vi "SpectraBinning.vi"(4 "BinType":T1, 5 "BinWidth":dbl=1.0, 7 "Binning":bool=TRUE, 8 "error in (no error)":errorcluster, 9 "Signal":dbl[](array[numeric]), 10 "m/z Array":dbl[](array[numeric]), 11 "GraphsRef.":refnum<vi>) -> (0 "error out":errorcluster, 2 "BinnedSpectrum":cluster{"m/z Array":dbl[], "Signal":dbl[]})   [LabVIEW 2012]
uses:
  BinType.ctl
  <vilib>/Analysis/baseanly.llb/Mean (DBL).vi
  <vilib>/Analysis/NI_AALBase.lvlib
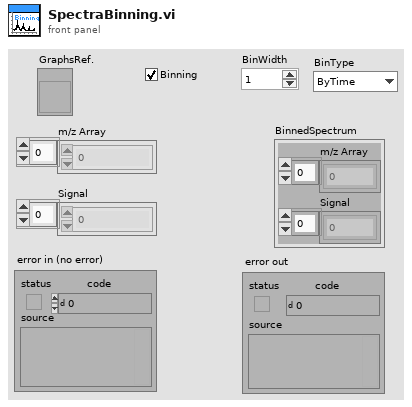
[diagram p1: front panel]
types:
  T1 = typedef "BinType.ctl" = enum16{"ByTime", "ByScreen", "ByMass", "ToUnitMass"}
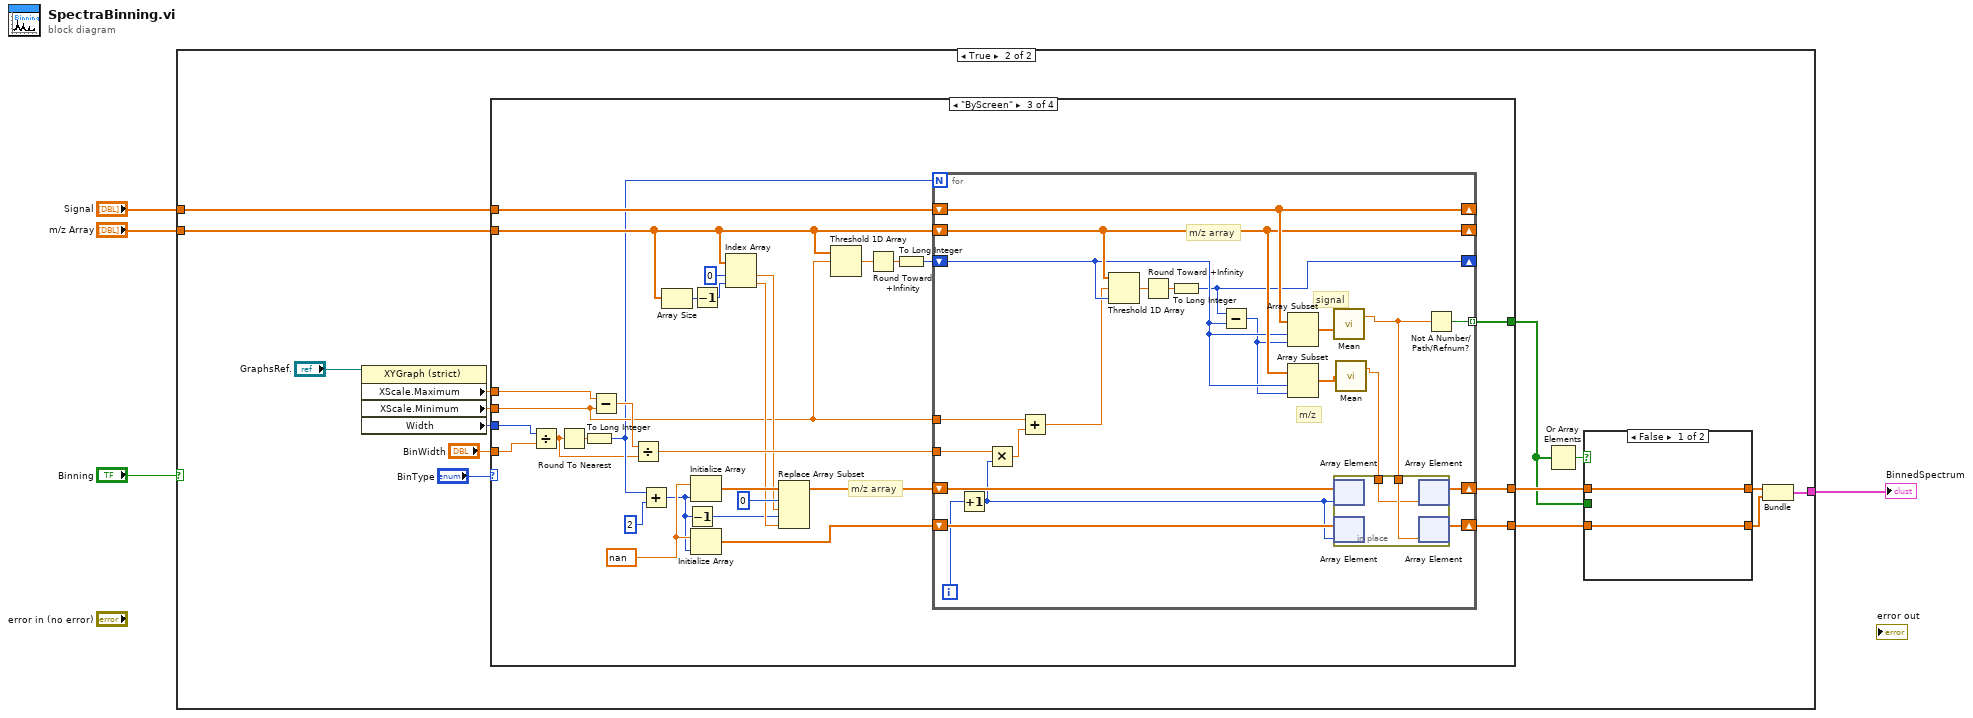
[diagram p0: block diagram]
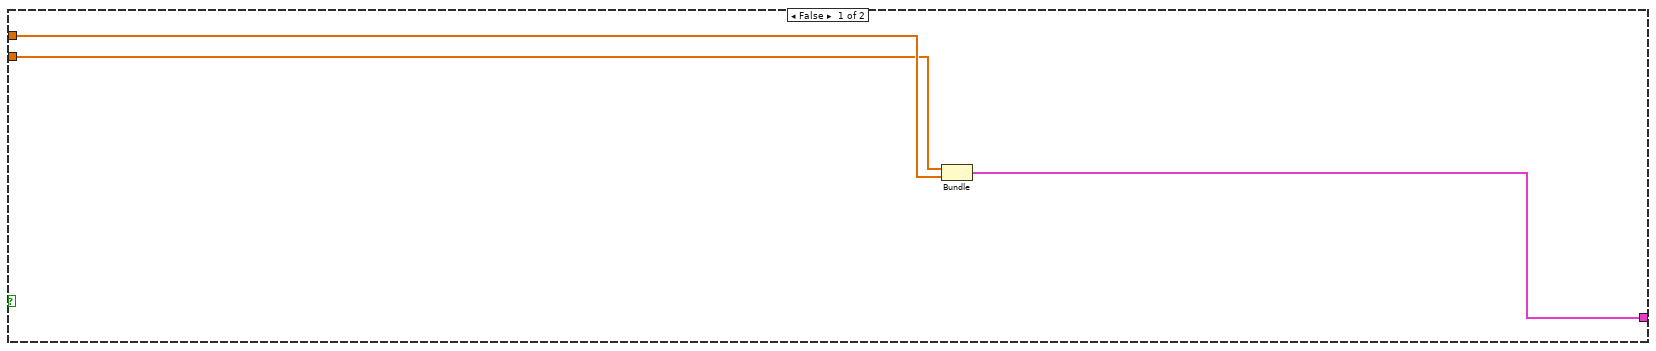
[diagram p2: hidden frame]
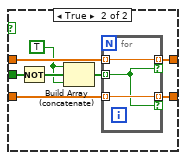
[diagram p3: hidden frame]
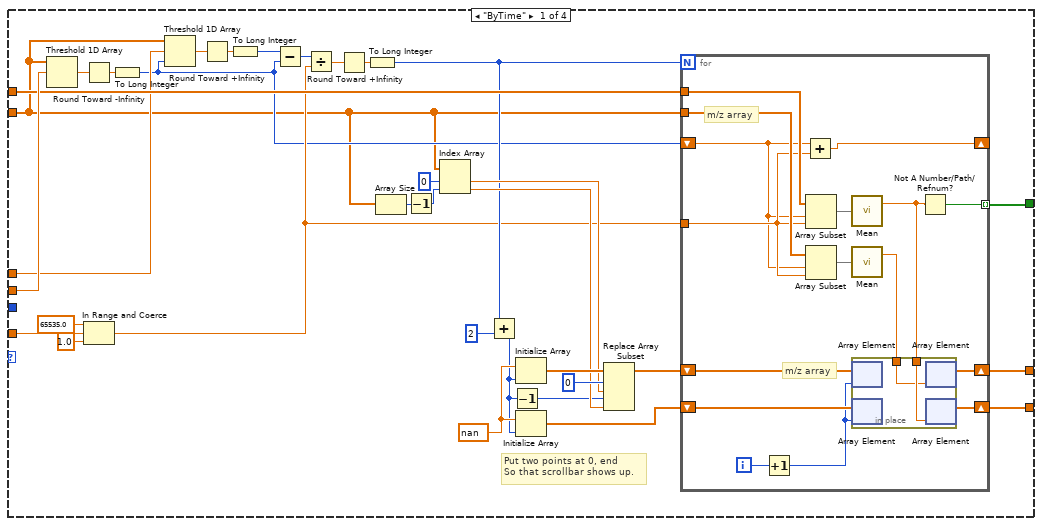
[diagram p4: hidden frame]
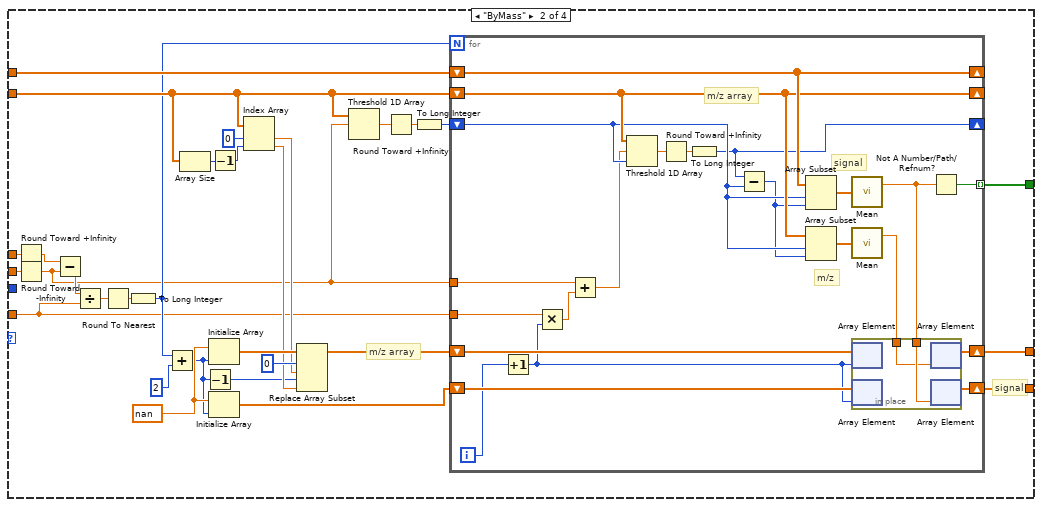
[diagram p5: hidden frame]
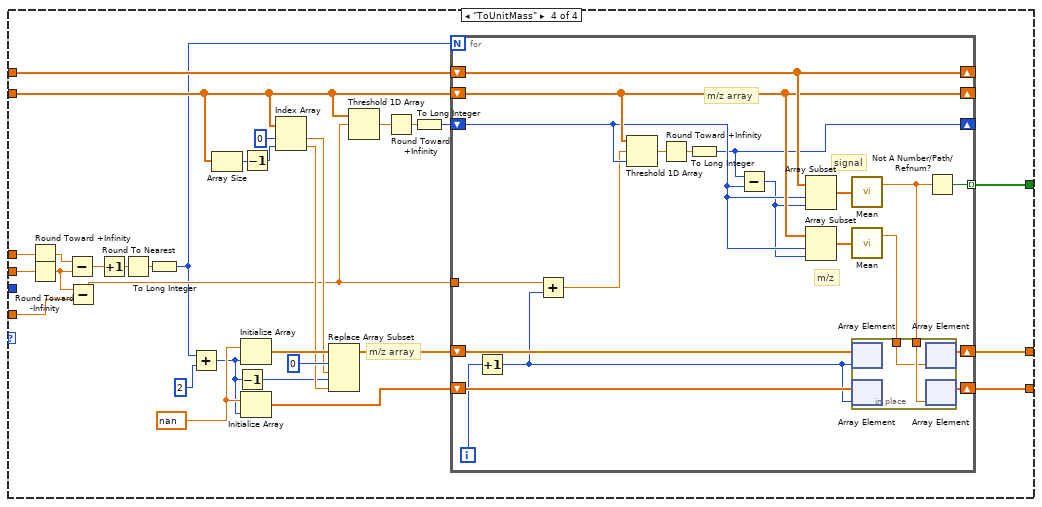
[diagram p6: hidden frame]
diagram:
  n1 = case shown="True" "Binning" {
    tunnel: [w7 w20] -> w4
    tunnel: "Signal" -> [w6 w10]
    tunnel: "m/z Array" -> [w5 w9]
    frame False {
      n2 = Bundle("m/z Array"=w5, "Signal"=w6) -> (w7:cluster{"m/z Array":dbl[], "Signal":dbl[]})  [unwired: 1 in]
    }
    frame True {
      n3 = property class="XYGraph (strict)"(reference="GraphsRef.") -> ("XScale.Maximum"=w13:dbl, "XScale.Minimum"=w12:dbl, "Width"=w11:u32)  [unwired: 1 in, 2 out]
      n4 = case shown="\"ByScreen\"" "BinType" {
        tunnel: w10 -> [w55 w117 w171 w226]
        tunnel: w9 -> [w36 w108 w160 w217]
        tunnel: w13 -> [w40 w102 w154 w211]
        tunnel: w12 -> [w56 w99 w150 w207]
        tunnel: w11 -> [_ _ w147 _]
        tunnel: "BinWidth" -> [w50 w95 w146 w199]
        tunnel: [w42 w90 w143 w197] -> w18
        tunnel: [w43 w89 w144 w198] -> w17
        tunnel: [w41 w91 w142 w196] -> w16
        frame "ByTime" {
          w67 = nan ("x/y")
          # "Put two points at 0, end\nSo that scrollbar shows up."
          n5 = Threshold 1D Array(2:w56, 3:w36) -> (0:w69:dbl)  [unwired: 1 in]
          n6 = Round Toward -Infinity(1:w69) -> (0:w68:dbl)
          n7 = In Range and Coerce(upper limit=65535.0, x=w50, lower limit=1.0) -> (coerced(x)=w46:dbl)  [unwired: 1 out]
          n8 = To Long Integer(number=w68) -> (32bit integer=w39:i32)
          n9 = Threshold 1D Array(1:w39, 2:w40, 3:w36) -> (0:w53:dbl)
          n10 = Round Toward +Infinity(x=w53) -> (ceil(x): smallest int >= x=w54:dbl)
          n11 = To Long Integer(number=w54) -> (32bit integer=w52:i32)
          n12 = Subtract(x=w52, y=w39) -> (x-y=w51:i32)
          n13 = Divide(x=w51, y=w46) -> (x/y=w48:dbl)
          n14 = Round Toward +Infinity(x=w48) -> (ceil(x): smallest int >= x=w49:dbl)
          n15 = To Long Integer(number=w49) -> (32bit integer=w47:i32)
          n16 = Array Size(array=w36) -> (size(s)=w59:i32)
          n17 = Decrement(x=w59) -> (x-1=w57:i32)
          n18 = Index Array(array=w36, index #1=0 ("index"), index #2=w57) -> (element #1=w61:dbl, element #2=w60:dbl)
          n19 = Add(x=w47, y=2) -> (x+y=w38:i32)
          n20 = Decrement(x=w38) -> (x-1=w58:i32)
          n21 = Initialize Array(w67, w38) -> (w66:dbl[])
          n22 = Initialize Array(w67, w38) -> (w65:dbl[])
          n23 = Replace Array Subset(array=w66, new element #1=w61, index #1=0 ("index"), new element #2=w60, index #2=w58) -> (w63:dbl[])
          n24 = for {
            N: w47 -> [_]
            shift-right: [w76] -> _
            shift-left: w39 -> [w74]
            shift-right: [w79] -> w43
            shift-left: w63 -> [w81]
            shift-right: [w78] -> w42
            shift-left: w65 -> [w80]
            tunnel: w46 -> [w75]
            tunnel: [w70] -> w41 mode=indexing
            tunnel: w36 -> [w82]
            tunnel: w55 -> [w85]
            i -> [w73]
            # "m/z array"
            # "m/z array"
            n25 = Increment(x=w73) -> (x+1=w72:i32)
            n26 = Add(x=w74, y=w75) -> (x+y=w76:dbl)
            n27 = Array Subset(array=w85, index=w74, length=w75) -> (w84:dbl[])
            n28 = Array Subset(array=w82, index=w74, length=w75) -> (w83:dbl[])
            n29 = call-poly <vilib>:"Mean.vi"("X"=w84) -> ("mean"=w71:dbl)  [unwired: 1 out]
            n30 = call-poly <vilib>:"Mean.vi"("X"=w83) -> ("mean"=w77:dbl)  [unwired: 1 out]
            n31 = in-place {
              in-place-border: w71 -> [w87]
              in-place-border: w77 -> [w86]
              n32 = in-place-array #1(w81, w72) -> ()  [unwired: 1 out]
              n33 = in-place-array #2(w80, w72) -> ()  [unwired: 1 out]
              n34 = in-place-array #1(w86) -> (w79:dbl[])  [unwired: 1 out]
              n35 = in-place-array #2(w87) -> (w78:dbl[])  [unwired: 1 out]
            }
            n36 = Not A Number/Path/Refnum?(number/path/refnum=w71) -> (NaN/Path/Refnum?=w70:bool)
          }
        }
        frame "ByMass" {
          w113 = nan ("x/y")
          # "signal"
          # "m/z array"
          n37 = Round Toward +Infinity(x=w102) -> (ceil(x): smallest int >= x=w92:dbl)
          n38 = Round Toward -Infinity(1:w99) -> (0:w93:dbl)
          n39 = Subtract(x=w92, y=w93) -> (x-y=w94:dbl)
          n40 = Divide(x=w94, y=w95) -> (x/y=w96:dbl)
          n41 = Round To Nearest(number=w96) -> (nearest integer value=w98:dbl)
          n42 = To Long Integer(number=w98) -> (32bit integer=w97:i32)
          n43 = Add(x=w97, y=2 ("x")) -> (x+y=w101:i32)
          n44 = Array Size(array=w108) -> (size(s)=w103:i32)
          n45 = Decrement(x=w101) -> (x-1=w88:i32)
          n46 = Initialize Array(w113, w101) -> (w112:dbl[])
          n47 = Initialize Array(w113, w101) -> (w111:dbl[])
          n48 = Decrement(x=w103) -> (x-1=w100:i32)
          n49 = Index Array(array=w108, index #1=0 ("index"), index #2=w100) -> (element #1=w105:dbl, element #2=w104:dbl)
          n50 = Replace Array Subset(array=w112, new element #1=w105, index #1=0 ("index"), new element #2=w104, index #2=w88) -> (w107:dbl[])
          n51 = Threshold 1D Array(2:w93, 3:w108) -> (0:w116:dbl)  [unwired: 1 in]
          n52 = Round Toward +Infinity(x=w116) -> (ceil(x): smallest int >= x=w115:dbl)
          n53 = To Long Integer(number=w115) -> (32bit integer=w114:i32)
          n54 = for {
            N: w97 -> [_]
            shift-right: [w139] -> _
            shift-left: w117 -> [w139]
            shift-right: [w136] -> _
            shift-left: w108 -> [w136]
            shift-right: [w126] -> _
            shift-left: w114 -> [w133]
            tunnel: w95 -> [w123]
            shift-right: [w129] -> w89
            shift-left: w107 -> [w131]
            shift-right: [w128] -> w90
            shift-left: w111 -> [w130]
            tunnel: w93 -> [w124]
            tunnel: [w120] -> w91 mode=indexing
            i -> [w118]
            # "signal"
            # "m/z"
            # "m/z array"
            n55 = Increment(x=w118) -> (x+1=w119:i32)
            n56 = Multiply(x=w123, y=w119) -> (x*y=w125:dbl)
            n57 = Add(x=w124, y=w125) -> (x+y=w127:dbl)
            n58 = Threshold 1D Array(1:w133, 2:w127, 3:w136) -> (0:w134:dbl)
            n59 = Round Toward +Infinity(x=w134) -> (ceil(x): smallest int >= x=w135:dbl)
            n60 = To Long Integer(number=w135) -> (32bit integer=w126:i32)
            n61 = Subtract(x=w126, y=w133) -> (x-y=w132:i32)
            n62 = Array Subset(array=w139, index=w133, length=w132) -> (w138:dbl[])
            n63 = Array Subset(array=w136, index=w133, length=w132) -> (w137:dbl[])
            n64 = call-poly <vilib>:"Mean.vi"("X"=w138) -> ("mean"=w121:dbl)  [unwired: 1 out]
            n65 = call-poly <vilib>:"Mean.vi"("X"=w137) -> ("mean"=w122:dbl)  [unwired: 1 out]
            n66 = in-place {
              in-place-border: w121 -> [w141]
              in-place-border: w122 -> [w140]
              n67 = in-place-array #3(w131, w119) -> ()  [unwired: 1 out]
              n68 = in-place-array #4(w130, w119) -> ()  [unwired: 1 out]
              n69 = in-place-array #3(w140) -> (w129:dbl[])  [unwired: 1 out]
              n70 = in-place-array #4(w141) -> (w128:dbl[])  [unwired: 1 out]
            }
            n71 = Not A Number/Path/Refnum?(number/path/refnum=w121) -> (NaN/Path/Refnum?=w120:bool)
          }
        }
        frame "ByScreen" {
          w165 = nan ("x/y")
          # "m/z array"
          n72 = Divide(x=w147, y=w146) -> (x/y=w145:dbl)
          n73 = Round To Nearest(number=w145) -> (nearest integer value=w149:dbl)
          n74 = To Long Integer(number=w149) -> (32bit integer=w148:i32)
          n75 = Subtract(x=w154, y=w150) -> (x-y=w169:dbl)
          n76 = Divide(x=w169, y=w145) -> (x/y=w166:dbl)
          n77 = Add(x=w148, y=2 ("x")) -> (x+y=w153:i32)
          n78 = Array Size(array=w160) -> (size(s)=w155:i32)
          n79 = Decrement(x=w153) -> (x-1=w152:i32)
          n80 = Initialize Array(w165, w153) -> (w164:dbl[])
          n81 = Initialize Array(w165, w153) -> (w163:dbl[])
          n82 = Decrement(x=w155) -> (x-1=w151:i32)
          n83 = Index Array(array=w160, index #1=0 ("index"), index #2=w151) -> (element #1=w157:dbl, element #2=w156:dbl)
          n84 = Replace Array Subset(array=w164, new element #1=w157, index #1=0 ("index"), new element #2=w156, index #2=w152) -> (w159:dbl[])
          n85 = Threshold 1D Array(2:w150, 3:w160) -> (0:w170:dbl)  [unwired: 1 in]
          n86 = Round Toward +Infinity(x=w170) -> (ceil(x): smallest int >= x=w168:dbl)
          n87 = To Long Integer(number=w168) -> (32bit integer=w167:i32)
          n88 = for {
            N: w148 -> [_]
            shift-right: [w193] -> _
            shift-left: w171 -> [w193]
            shift-right: [w192] -> _
            shift-left: w160 -> [w192]
            shift-right: [w181] -> _
            shift-left: w167 -> [w189]
            tunnel: w166 -> [w177]
            shift-right: [w184] -> w144
            shift-left: w159 -> [w187]
            shift-right: [w183] -> w143
            shift-left: w163 -> [w186]
            tunnel: w150 -> [w178]
            tunnel: [w176] -> w142 mode=indexing
            i -> [w185]
            # "signal"
            # "m/z"
            # "m/z array"
            n89 = Increment(x=w185) -> (x+1=w180:i32)
            n90 = Multiply(x=w177, y=w180) -> (x*y=w179:dbl)
            n91 = Add(x=w178, y=w179) -> (x+y=w182:dbl)
            n92 = Threshold 1D Array(1:w189, 2:w182, 3:w192) -> (0:w190:dbl)
            n93 = Round Toward +Infinity(x=w190) -> (ceil(x): smallest int >= x=w191:dbl)
            n94 = To Long Integer(number=w191) -> (32bit integer=w181:i32)
            n95 = Subtract(x=w181, y=w189) -> (x-y=w188:i32)
            n96 = Array Subset(array=w193, index=w189, length=w188) -> (w173:dbl[])
            n97 = Array Subset(array=w192, index=w189, length=w188) -> (w175:dbl[])
            n98 = call-poly <vilib>:"Mean.vi"("X"=w173) -> ("mean"=w172:dbl)  [unwired: 1 out]
            n99 = call-poly <vilib>:"Mean.vi"("X"=w175) -> ("mean"=w174:dbl)  [unwired: 1 out]
            n100 = in-place {
              in-place-border: w172 -> [w195]
              in-place-border: w174 -> [w194]
              n101 = in-place-array #5(w187, w180) -> ()  [unwired: 1 out]
              n102 = in-place-array #6(w186, w180) -> ()  [unwired: 1 out]
              n103 = in-place-array #5(w194) -> (w184:dbl[])  [unwired: 1 out]
              n104 = in-place-array #6(w195) -> (w183:dbl[])  [unwired: 1 out]
            }
            n105 = Not A Number/Path/Refnum?(number/path/refnum=w172) -> (NaN/Path/Refnum?=w176:bool)
          }
        }
        frame "ToUnitMass" {
          w222 = nan ("x/y")
          # "m/z array"
          n106 = Round Toward +Infinity(x=w211) -> (ceil(x): smallest int >= x=w205:dbl)
          n107 = Round Toward -Infinity(1:w207) -> (0:w206:dbl)
          n108 = Subtract(x=w205, y=w206) -> (x-y=w204:dbl)
          n109 = Subtract(x=w206, y=w199) -> (x-y=w202:dbl)
          n110 = Increment(x=w204) -> (x+1=w203:dbl)
          n111 = Round To Nearest(number=w203) -> (nearest integer value=w201:dbl)
          n112 = To Long Integer(number=w201) -> (32bit integer=w200:i32)
          n113 = Add(x=w200, y=2 ("x")) -> (x+y=w210:i32)
          n114 = Array Size(array=w217) -> (size(s)=w212:i32)
          n115 = Decrement(x=w210) -> (x-1=w209:i32)
          n116 = Initialize Array(w222, w210) -> (w221:dbl[])
          n117 = Initialize Array(w222, w210) -> (w220:dbl[])
          n118 = Decrement(x=w212) -> (x-1=w208:i32)
          n119 = Index Array(array=w217, index #1=0 ("index"), index #2=w208) -> (element #1=w214:dbl, element #2=w213:dbl)
          n120 = Replace Array Subset(array=w221, new element #1=w214, index #1=0 ("index"), new element #2=w213, index #2=w209) -> (w216:dbl[])
          n121 = Threshold 1D Array(2:w202, 3:w217) -> (0:w225:dbl)  [unwired: 1 in]
          n122 = Round Toward +Infinity(x=w225) -> (ceil(x): smallest int >= x=w224:dbl)
          n123 = To Long Integer(number=w224) -> (32bit integer=w223:i32)
          n124 = for {
            N: w200 -> [_]
            shift-right: [w246] -> _
            shift-left: w226 -> [w246]
            shift-right: [w243] -> _
            shift-left: w217 -> [w243]
            shift-right: [w232] -> _
            shift-left: w223 -> [w240]
            shift-right: [w235] -> w198
            shift-left: w216 -> [w238]
            shift-right: [w234] -> w197
            shift-left: w220 -> [w237]
            tunnel: w202 -> [w231]
            tunnel: [w227] -> w196 mode=indexing
            i -> [w236]
            # "signal"
            # "m/z"
            # "m/z array"
            n125 = Increment(x=w236) -> (x+1=w229:i32)
            n126 = Add(x=w231, y=w229) -> (x+y=w233:dbl)
            n127 = Threshold 1D Array(1:w240, 2:w233, 3:w243) -> (0:w241:dbl)
            n128 = Round Toward +Infinity(x=w241) -> (ceil(x): smallest int >= x=w242:dbl)
            n129 = To Long Integer(number=w242) -> (32bit integer=w232:i32)
            n130 = Subtract(x=w232, y=w240) -> (x-y=w239:i32)
            n131 = Array Subset(array=w246, index=w240, length=w239) -> (w245:dbl[])
            n132 = Array Subset(array=w243, index=w240, length=w239) -> (w244:dbl[])
            n133 = call-poly <vilib>:"Mean.vi"("X"=w245) -> ("mean"=w228:dbl)  [unwired: 1 out]
            n134 = call-poly <vilib>:"Mean.vi"("X"=w244) -> ("mean"=w230:dbl)  [unwired: 1 out]
            n135 = in-place {
              in-place-border: w228 -> [w248]
              in-place-border: w230 -> [w247]
              n136 = in-place-array #7(w238, w229) -> ()  [unwired: 1 out]
              n137 = in-place-array #8(w237, w229) -> ()  [unwired: 1 out]
              n138 = in-place-array #7(w247) -> (w235:dbl[])  [unwired: 1 out]
              n139 = in-place-array #8(w248) -> (w234:dbl[])  [unwired: 1 out]
            }
            n140 = Not A Number/Path/Refnum?(number/path/refnum=w228) -> (NaN/Path/Refnum?=w227:bool)
          }
        }
      }
      n141 = Or Array Elements(Boolean array=w16) -> (logical OR=w19:bool)
      n142 = case shown="False" w19 {
        tunnel: [w24 w32] -> w15
        tunnel: w17 -> [w24 w31]
        tunnel: [w23 w30] -> w14
        tunnel: w18 -> [w23 w29]
        tunnel: w16 -> [_ w28]
        frame False {
        }
        frame True {
          w25 = TRUE
          n143 = Not(x=w28) -> (.not. x?=w26:bool[])
          n144 = Build Array (concatenate)(w25, w26, w25) -> (w27:bool[])
          n145 = for {
            tunnel: [w35] -> w32 mode=indexing if=w33
            tunnel: w31 -> [w35] mode=indexing
            tunnel: [w34] -> w30 mode=indexing if=w33
            tunnel: w29 -> [w34] mode=indexing
            tunnel: w27 -> [w33] mode=indexing
          }
        }
      }
      n146 = Bundle(w15, w14) -> (w20:cluster{dbl[], dbl[]})  [unwired: 1 in]
    }
  }
  "BinnedSpectrum" <- w4
